vi "Write Configuration (INI) File.vi"(8 "error in":errorcluster) -> (0 "error out":errorcluster)   [LabVIEW 2017]
doc: "Illustrates how to create and write a configuration settings file. Enter values in the controls on the front panel then click on the Run Arrow. To read the file, run Read Configuration (INI) File.vi."
uses:
  <vilib>/Utility/config.llb/Read Key (String).vi
  <vilib>/Utility/config.llb/Write Key (String).vi
  <vilib>/Utility/config.llb/NI_LVConfig.lvlib
panel:
  in  "Cancel Button":bool
  in  "Save Button":bool
  in  "Encoder Resolution":string
  in  "Error Speed":string
  in  "Error Current":string
  in  "Error Position":string
  in  "Firmware Version":string
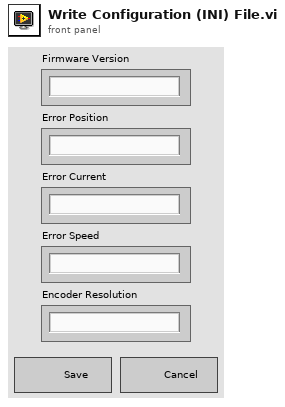
[diagram p1: front panel]
types:
  T1 = typedef "NI_LVConfig.lvlib/Config Data RefNum.ctl" = refnum<k1>
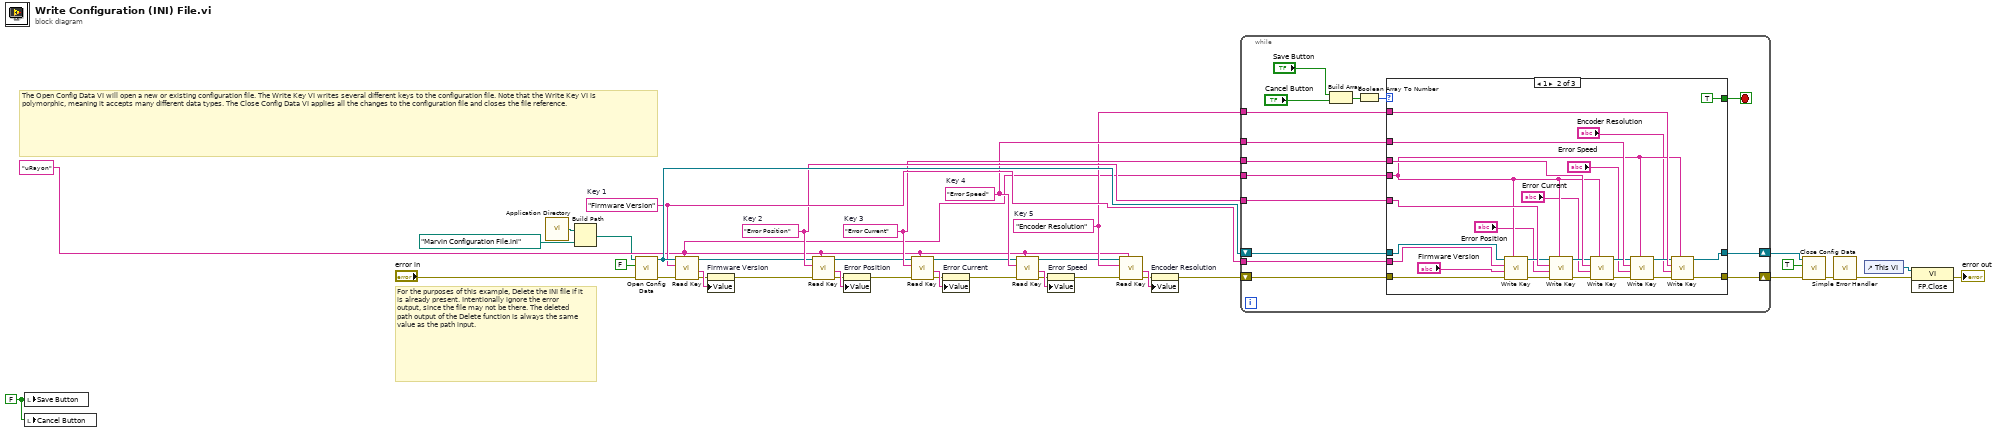
[diagram p0: block diagram]
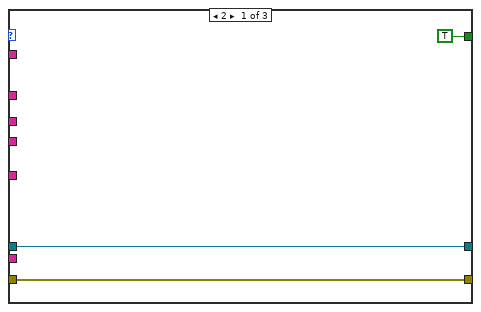
[diagram p2: hidden frame]
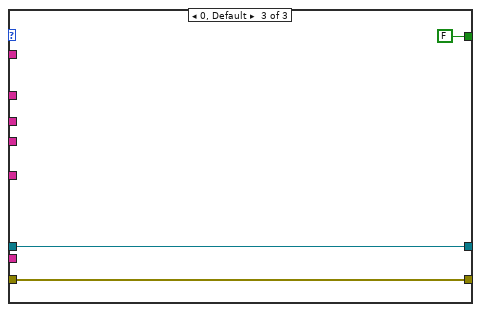
[diagram p3: hidden frame]
diagram:
  w1 = FALSE ("Save Button")
  w32 = "Encoder Resolution"  # Key 5
  w33 = "Error Speed"  # Key 4
  w34 = "Error Current"  # Key 3
  w35 = "Error Position"  # Key 2
  w36 = "Firmware Version"  # Key 1
  w28 = "uRayon"
  # "The Open Config Data VI will open a new or existing configuration file. The Write Key VI writes several different keys to the configuration file. Note that the Write Key VI is polymorphic, meaning it accepts many different data types. The Close Config Data VI applies all the changes to the configuration file and closes the file reference."
  # "For the purposes of this example, Delete the INI file if it is already present. Intentionally ignore the error output, since the file may not be there. The deleted path output of the Delete function is always the same value as the path input."
  n1 = local write "Save Button"(w1) -> ()
  n2 = local write "Cancel Button"(w1) -> ()
  n3 = call <vilib>:"Application Directory.vi"() -> ("Application Directory"=w29:path)
  n4 = Build Path(base path=w29, name or relative path=path "Marvin Configuration File.ini" ("default name")) -> (appended path=w3:path)
  n5 = call <vilib>:"Open Config Data.vi"("error in (no error)"="error in", "create file if necessary (T)"=FALSE, "configuration file path"=w3) -> ("error out"=w38:errorcluster, "refnum"=w40:T1)  [unwired: 7 out]
  n6 = call-poly <vilib>:"Read Key.vi"("section"=w28, "error in (no error)"=w38, "key"=w36, "refnum"=w40) -> ("error out"=w22:errorcluster, "value"=w23:string, "refnum out"=w21:T1)  [unwired: 2 in, 3 out]
  n7 = property on="Firmware Version" class="Str"(error in=w22, "Value"=w23) -> (error out=w17:errorcluster)  [unwired: 1 in, 1 out]
  n8 = call-poly <vilib>:"Read Key.vi"("section"=w28, "error in (no error)"=w17, "key"=w35, "refnum"=w21) -> ("error out"=w15:errorcluster, "value"=w16:string, "refnum out"=w20:T1)  [unwired: 2 in, 3 out]
  n9 = property on="Error Position" class="Str"(error in=w15, "Value"=w16) -> (error out=w14:errorcluster)  [unwired: 1 in, 1 out]
  n10 = call-poly <vilib>:"Read Key.vi"("section"=w28, "error in (no error)"=w14, "key"=w34, "refnum"=w20) -> ("error out"=w12:errorcluster, "value"=w13:string, "refnum out"=w19:T1)  [unwired: 2 in, 3 out]
  n11 = property on="Error Current" class="Str"(error in=w12, "Value"=w13) -> (error out=w11:errorcluster)  [unwired: 1 in, 1 out]
  n12 = call-poly <vilib>:"Read Key.vi"("section"=w28, "error in (no error)"=w11, "key"=w33, "refnum"=w19) -> ("error out"=w9:errorcluster, "value"=w10:string, "refnum out"=w18:T1)  [unwired: 2 in, 3 out]
  n13 = property on="Error Speed" class="Str"(error in=w9, "Value"=w10) -> (error out=w8:errorcluster)  [unwired: 1 in, 1 out]
  n14 = call-poly <vilib>:"Read Key.vi"("section"=w28, "error in (no error)"=w8, "key"=w32, "refnum"=w18) -> ("error out"=w6:errorcluster, "value"=w7:string)  [unwired: 2 in, 4 out]
  n15 = property on="Encoder Resolution" class="Str"(error in=w6, "Value"=w7) -> (error out=w5:errorcluster)  [unwired: 1 in, 1 out]
  n16 = while {
    tunnel: w36 -> [w52]
    tunnel: w35 -> [w51]
    tunnel: w34 -> [w50]
    tunnel: w33 -> [w49]
    tunnel: w32 -> [w48]
    tunnel: w28 -> [w47]
    shift-right: [w54] -> w39
    shift-left: w40 -> [w55]
    shift-right: [w53] -> w37
    shift-left: w5 -> [w46]
    stop <- w42 stop-if-true
    n17 = Build Array("Save Button", "Cancel Button") -> (w43:bool[])
    n18 = Boolean Array To Number(Boolean array=w43) -> (number=w41:u32)
    n19 = case shown="1" w41 {
      tunnel: w55 -> [w58 w82 w84]
      tunnel: [w58 w81 w84] -> w54
      tunnel: [w57 w80 w83] -> w53
      tunnel: w52 -> [_ w79 _]
      tunnel: w51 -> [_ w78 _]
      tunnel: w50 -> [_ w77 _]
      tunnel: w49 -> [_ w76 _]
      tunnel: w48 -> [_ w75 _]
      tunnel: w47 -> [_ w74 _]
      tunnel: w46 -> [w57 w60 w83]
      tunnel: [TRUE TRUE FALSE] -> w42
      frame 2 {
      }
      frame 1 {
        n20 = call-poly <vilib>:"Write Key.vi"("section"=w74, "error in (no error)"=w60, "value"="Firmware Version", "key"=w79, "refnum"=w82) -> ("error out"=w69:errorcluster, "refnum out"=w73:T1)  [unwired: 1 in, 4 out]
        n21 = call-poly <vilib>:"Write Key.vi"("section"=w74, "error in (no error)"=w69, "value"="Error Position", "key"=w78, "refnum"=w73) -> ("error out"=w68:errorcluster, "refnum out"=w72:T1)  [unwired: 1 in, 4 out]
        n22 = call-poly <vilib>:"Write Key.vi"("section"=w74, "error in (no error)"=w68, "value"="Error Current", "key"=w77, "refnum"=w72) -> ("error out"=w67:errorcluster, "refnum out"=w71:T1)  [unwired: 1 in, 4 out]
        n23 = call-poly <vilib>:"Write Key.vi"("section"=w74, "error in (no error)"=w67, "value"="Error Speed", "key"=w76, "refnum"=w71) -> ("error out"=w66:errorcluster, "refnum out"=w70:T1)  [unwired: 1 in, 4 out]
        n24 = call-poly <vilib>:"Write Key.vi"("section"=w74, "error in (no error)"=w66, "value"="Encoder Resolution", "key"=w75, "refnum"=w70) -> ("error out"=w80:errorcluster, "refnum out"=w81:T1)  [unwired: 1 in, 4 out]
      }
      frame 0, Default {
      }
    }
  }
  n25 = call <vilib>:"Close Config Data.vi"("error in (no error)"=w37, "write file if changed (T)"=TRUE, "refnum"=w39) -> ("error out"=w31:errorcluster)  [unwired: 8 out]
  n26 = call <vilib>:"Simple Error Handler.vi"("error in (no error)"=w31) -> ("error out"=w26:errorcluster)  [unwired: 1 in, 7 out]
  n27 = control-ref of="This VI"() -> (w27:refnum<vi>)
  n28 = invoke class="VI" method="FP.Close"(reference=w27, error in=w26) -> (error out=→"error out":errorcluster)  [unwired: 1 in, 2 out]
